vi "I2Csetpixels.vi"(0 "I2C Reference In":string, 1 "Color Box - On":u32, 5 "Brightness (0-255)":u8, 9 "LED Position":u8, 11 "Error In":errorcluster, 12 "Color Box - Off":u32) -> (4 "I2C Reference Out":T1 {"Device Address" format="%.0x"}, 15 "Error Out":errorcluster)   [LabVIEW 2015]
uses:
  <vilib>/Rock Robotics/WPI/I2C/WPI_I2CDevRef.ctl
  <vilib>/Rock Robotics/SystemInterfaces/i2clib/i2c_bus.ctl
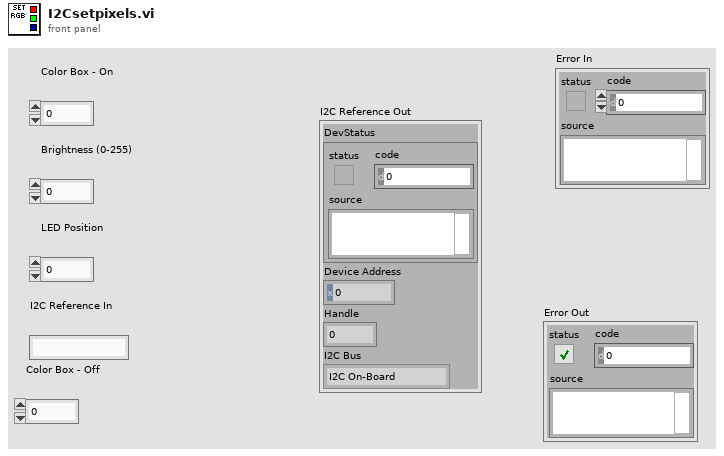
[diagram p1: front panel]
types:
  T1 = typedef "WPI_I2CDevRef.ctl" = cluster{"DevStatus":errorcluster, "Device Address":u8, "Handle":i32, "I2C Bus":T2}
  T2 = typedef "i2c_bus.ctl" = enum16{"I2C On-Board", "I2C MXP", "Invalid"}
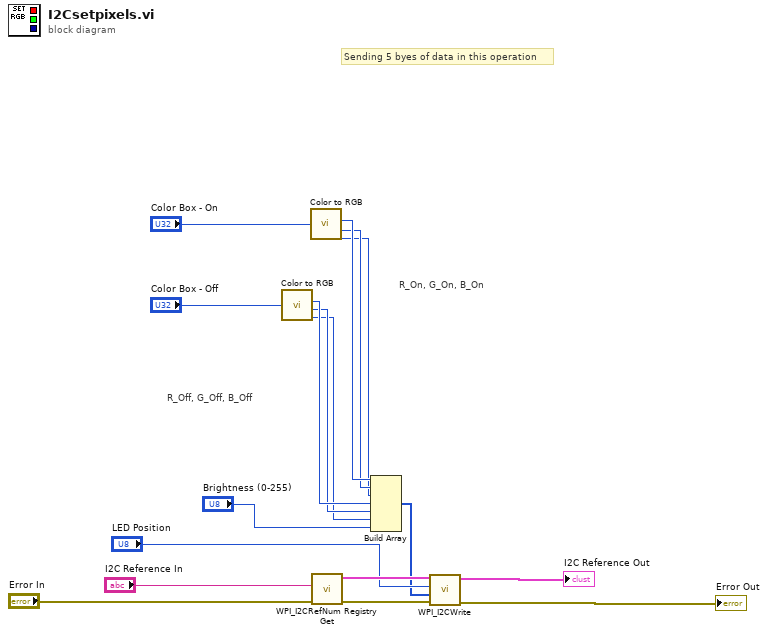
[diagram p0: block diagram]
diagram:
  # "R_Off, G_Off, B_Off"
  # "R_On, G_On, B_On"
  # "Sending 5 byes of data in this operation"
  n1 = call <vilib>:"Color to RGB.vi"("Color"="Color Box - Off") -> ("R"=w3:u8, "G"=w2:u8, "B"=w1:u8)  [unwired: 1 out]
  n2 = call <vilib>:"Color to RGB.vi"("Color"="Color Box - On") -> ("R"=w13:u8, "G"=w7:u8, "B"=w6:u8)  [unwired: 1 out]
  n3 = call <vilib>:"WPI_I2CRefNum Registry Get.vi"("error in (no error)"="Error In", "refnum name"="I2C Reference In") -> ("error out"=w17:errorcluster, "I2CDevRef"=w16:T1)  [unwired: 8 in]
  n4 = Build Array(w13, w7, w6, w3, w2, w1, "Brightness (0-255)") -> (w14:u8[])
  n5 = call <vilib>:"WPI_I2CWrite.vi"("error in (no error)"=w17, "I2CDataToSend"=w14, "I2CRegister"="LED Position", "I2CDevRef"=w16) -> ("error out"=→"Error Out":errorcluster, "I2CDevRef"=→"I2C Reference Out":T1)  [unwired: 6 in]
